vi "Custom Command.vi"(7 "Timeout (100 ms)":i32=100, 8 "Error In":errorcluster, 9 "Data":u8[](array[numeric]), 10 "Custom Command Number":u16, 11 "LINX Resource":T1) -> (0 "Error Out":errorcluster, 1 "Response":u8[](array[numeric]), 2 "Dup Command Number":u16, 3 "LINX Resource":T1)   [LabVIEW 2011, in "LVH-LINX.lvlib"]
doc: "Call a custom command in the LINX firmware. You must add the custom command to the LINX firmware before you are able to call it using this VI. Use this VI to access advanced functionality that must execute on the device.\n\nThe timeout value indicates how long LabVIEW will wait for the custom command to complete. Set this value slightly higher than the expected time required for the custom function to complete. This VI will wait up to the time specified in timeout, and will rseturn as soon as the function is complete."
uses:
  LVH-LINX.lvlib
  Private/Type Defs/LINX Ref.ctl
  Private/Type Defs/Platform.ctl
  Private/Type Defs/Interface.ctl
  Private/Device/Type Defs/LINX Device Config.ctl
  Private/Device/Type Defs/TCP Config.ctl
  Private/Device/Type Defs/Channels.ctl
  Private/Type Defs/Error Type.ctl
  Private/Device/Device.lvlib
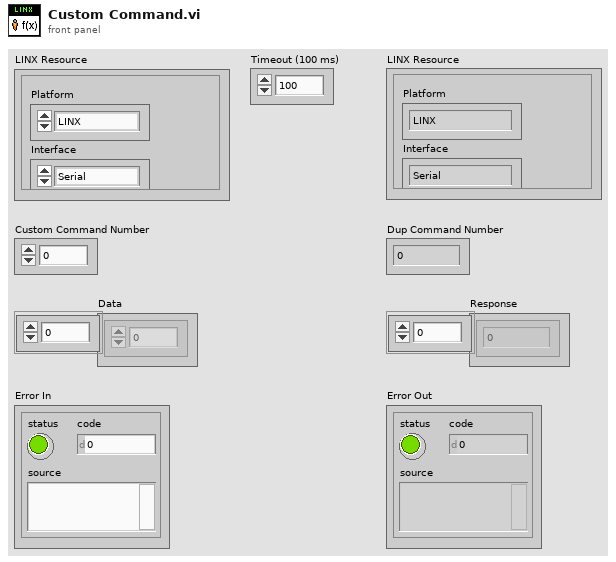
[diagram p1: front panel]
types:
  T1 = typedef "LVH-LINX.lvlib/LINX Ref.ctl" = cluster{"Platform":T2, "Interface":T3, "LINX Device Config":T4}
  T2 = typedef "LVH-LINX.lvlib/Platform.ctl" = enum16{"LINX", "myRIO"}
  T3 = typedef "LVH-LINX.lvlib/Interface.ctl" = enum16{"Serial", "TCP"}
  T4 = typedef "LVH-LINX.lvlib/Device.lvlib/LINX Device Config.ctl" = cluster{"Interface":T3, "COM Port":refnum<visa-resource-name>, "TCP Configuration":T5, "Device Family":u8, "Device ID":u8, "Device Name":string, "TCP Ref":refnum<k5>, "Channels":T6}
  T5 = typedef "LVH-LINX.lvlib/Device.lvlib/TCP Config.ctl" = cluster{"IP Address":string, "Port":u16}
  T6 = typedef "LVH-LINX.lvlib/Channels.ctl" = cluster{"DI Channels":u8[], "DO Channels":u8[], "AI":u8[], "AO":u8[], "PWM":u8[], "QE":u8[], "UART":u8[], "I2C 2":u8[], "SPI":u8[], "CAN":u8[], "AI Ref (V)":dbl, "AO Resolution (Bits)":u8, "AO Ref (V)":dbl}
  T7 = typedef "LVH-LINX.lvlib/Error Type.ctl" = enum16{"Unknown", "Timeout", "Corrupt Return Packet", "Unable To Connect", "Command Not Supported", "Channel DNE", "Invalid COM Config", "Firmware Version Mismatch", "myRIO Support"}
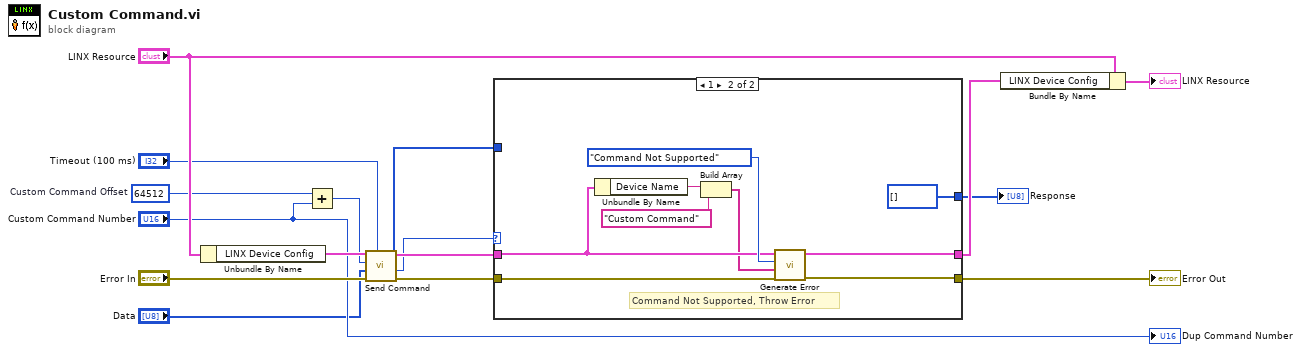
[diagram p0: block diagram]
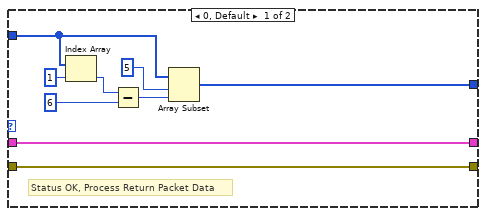
[diagram p2: hidden frame]
diagram:
  w6 = u16 64512  # Custom Command Offset
  n1 = Unbundle By Name("LINX Resource") -> ("LINX Device Config"=w9:T4)
  n2 = Add(x=w6, y="Custom Command Number") -> (x+y=w5:u16)
  n3 = call "Send Command.vi"("Timeout (100 ms)"="Timeout (100 ms)", "Error In"="Error In", "ARGS"="Data", "CMD"=w5, "LINX Device Config"=w9) -> ("Error Out"=w12:errorcluster, "Status"=w7:u8, "Response"=w11:u8[], "LINX Device Config"=w14:T4)  [unwired: 3 in]
  n4 = case shown="1" w7 {
    tunnel: [w25 w32] -> w10
    tunnel: w14 -> [w25 w29]
    tunnel: [w24 w33] -> w13
    tunnel: w12 -> [w24 w34]
    tunnel: w11 -> [w19 _]
    tunnel: [w17 u8[] [] ("Response")] -> w2
    frame 0, Default {
      # "Status OK, Process Return Packet Data"
      n5 = Index Array(array=w19, index=1) -> (element=w22:u8)
      n6 = Subtract(x=w22, y=u8 6) -> (x-y=w20:u8)
      n7 = Array Subset(array=w19, index=5, length=w20) -> (w17:u8[])
    }
    frame 1 {
      # "Command Not Supported, Throw Error"
      n8 = Unbundle By Name(w29) -> ("Device Name"=w30:string)
      n9 = Build Array(w30, "Custom Command" ("element")) -> (w28:string[])
      n10 = call "Generate Error.vi"("Error In"=w34, "Arguments"=w28, "Error Type"=Error_Type."Command Not Supported", "LINX Device Config"=w29) -> ("Error Out"=w33:errorcluster, "LINX Device Config"=w32:T4)  [unwired: 6 in]
    }
  }
  "Error Out" <- w13
  "Response" <- w2
  n11 = Bundle By Name(cluster="LINX Resource", "LINX Device Config"=w10) -> (→"LINX Resource":T1)
  "Dup Command Number" <- "Custom Command Number"
